vi "Relay - cycle.vi"(8 "error in":errorcluster, 9 "switch time":dbl[unit]=0.01, 10 "pulse length":dbl[unit]=0.05, 11 "task in":refnum<k21>) -> (0 "error out":errorcluster, 3 "task out":refnum<k21>)   [LabVIEW 2009]
doc: "Cycles one output on and then off, using timing information supplied. Used to control a relay while switching between different resonant circuits (to resonate the nuclei more effectively)."
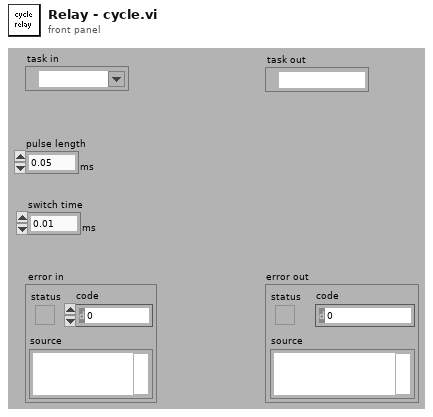
[diagram p1: front panel]
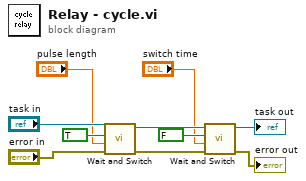
[diagram p0: block diagram]
diagram:
  n1 = call "Wait and Switch.vi"("error in"="error in", "Wait for"="pulse length", "Switch to"=TRUE, "task in"="task in") -> ("error out"=w7:errorcluster, "task out"=w6:refnum<k21>)  [unwired: 6 out]
  n2 = call "Wait and Switch.vi"("error in"=w7, "Wait for"="switch time", "Switch to"=FALSE, "task in"=w6) -> ("error out"=→"error out":errorcluster, "task out"=→"task out":refnum<k21>)  [unwired: 6 out]
